vi "BuyProductSabritas.vi"(8 "error in (no error)":errorcluster, 10 "Description":T1, 11 "UI Actor in":refnum<class "UI Actor.lvclass">) -> (0 "error out":errorcluster, 3 "UI Actor out":refnum<class "UI Actor.lvclass">)   [LabVIEW 2020, in "UI Actor.lvlib" / "UI Actor.lvclass"]
uses:
  UI Actor.lvclass
  UI Actor.lvclass/UI Actor.ctl
  ESP Actor Messages/Update MSG Msg/Update MSG Msg.lvclass/Update MSG Msg.ctl
  <vilib>/ActorFramework/Message Enqueuer/Message Enqueuer.lvclass/Message Enqueuer.ctl
  <vilib>/ActorFramework/Message Enqueuer/Enqueue.vi
  ESP Actor Messages/Update MSG Msg/Update MSG Msg.lvclass
  C:/Program Files (x86)/National Instruments/LabVIEW 2020/vi.lib/ActorFramework/Message/Message.lvclass
  Sabritas Actor Messages/UpdateInventorySabritas Msg/UpdateInventorySabritas Msg.lvclass
  <vilib>/Utility/config.llb/Write Key (I32).vi
  <vilib>/ActorFramework/Message Priority Queue/Priority Enqueue.vi
  <vilib>/Utility/config.llb/NI_LVConfig.lvlib
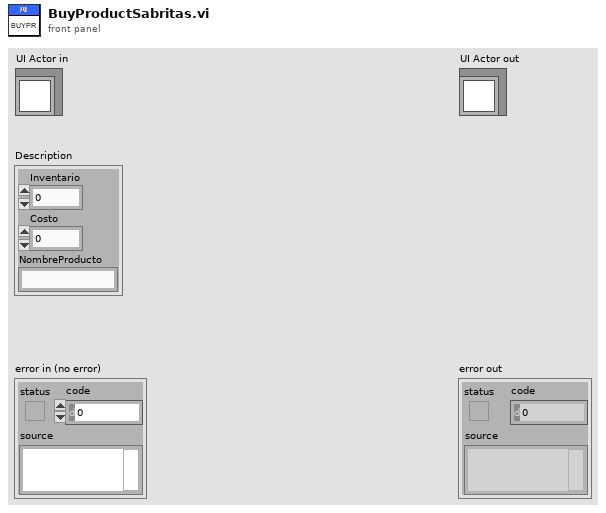
[diagram p1: front panel]
types:
  T1 = cluster{"Inventario":i32, "Costo":dbl, "NombreProducto":string}
  T2 = typedef "NI_LVConfig.lvlib/Config Data RefNum.ctl" = refnum<k1>
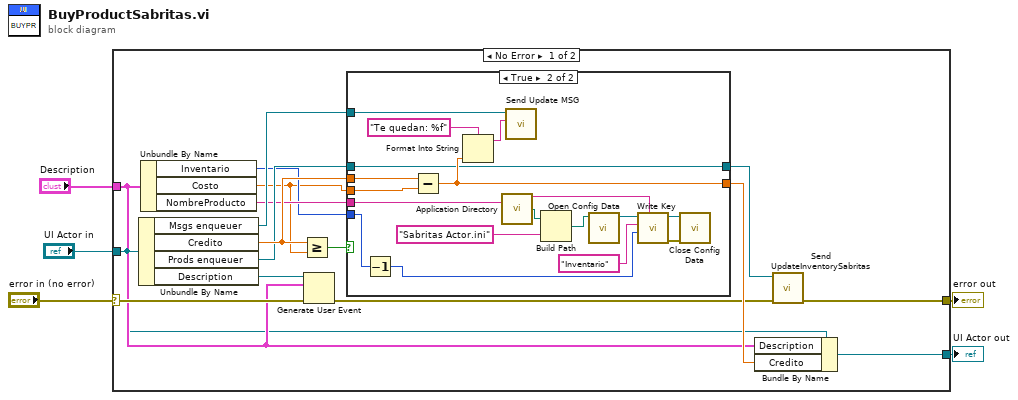
[diagram p0: block diagram]
diagram:
  n1 = case shown="No Error" "error in (no error)" {
    selector: "error in (no error)" -> [w12 w42]
    tunnel: [w8 w42] -> w4
    tunnel: [w11 w41] -> w2
    tunnel: "UI Actor in" -> [w6 w41]
    tunnel: "Description" -> [w10 _]
    frame No Error {
      n2 = Unbundle By Name(w6) -> ("Msgs enqueuer"=w18:refnum<class "Message Enqueuer.lvclass">, "Credito"=w19:dbl, "Prods enqueuer"=w16:refnum<class "Message Enqueuer.lvclass">, "Description"=w20:refnum<user-event>)
      n3 = Unbundle By Name(w10) -> ("Inventario"=w14:i32, "Costo"=w13:dbl, "NombreProducto"=w15:string)
      n4 = Greater Or Equal?(x=w19, y=w13) -> (x >= y?=w21:bool)
      n5 = Generate User Event(user event=w20, event data cluster=w10, error in=w12) -> (error out=w9:errorcluster)  [unwired: 1 in, 1 out]
      n6 = case shown="True" w21 {
        tunnel: w19 -> [w23 w40]
        tunnel: w18 -> [_ w37]
        tunnel: [w23 w36] -> w17
        tunnel: w16 -> [w22 w27]
        tunnel: [w22 w27] -> w7
        tunnel: w15 -> [_ w26]
        tunnel: w14 -> [_ w25]
        tunnel: w13 -> [_ w24]
        frame False {
        }
        frame True {
          n7 = Decrement(x=w25) -> (x-1=w32:i32)
          n8 = Subtract(x=w40, y=w24) -> (x-y=w36:dbl)
          n9 = Format Into String(format string="Te quedan: %f", w36) -> (resulting string=w38:string)  [unwired: 2 in, 1 out]
          n10 = call <vilib>:"Application Directory.vi"() -> ("Application Directory"=w35:path)
          n11 = call "Send Update MSG.vi"("Update MSG"=w38, "Message Enqueuer"=w37) -> ()  [unwired: 8 in, 2 out]
          n12 = Build Path(base path=w35, name or relative path="Sabritas Actor.ini") -> (appended path=w34:path)
          n13 = call <vilib>:"Open Config Data.vi"("configuration file path"=w34) -> ("refnum"=w33:T2)  [unwired: 8 in, 2 out]
          n14 = call-poly <vilib>:"Write Key.vi"("section"=w26, "value"=w32, "key"="Inventario", "refnum"=w33) -> ("error out"=w29:errorcluster, "refnum out"=w30:T2)  [unwired: 5 in, 1 out]
          n15 = call <vilib>:"Close Config Data.vi"("error in (no error)"=w29, "refnum"=w30) -> ()  [unwired: 8 in, 2 out]
        }
      }
      n16 = Bundle By Name(cluster=w6, "Description"=w10, "Credito"=w17) -> (w11:refnum<class "UI Actor.lvclass">)
      n17 = call "Send UpdateInventorySabritas.vi"("error in (no error)"=w9, "Message Enqueuer"=w7) -> ("error out"=w8:errorcluster)  [unwired: 8 in, 1 out]
    }
    frame Error {
    }
  }
  "error out" <- w4
  "UI Actor out" <- w2
